vi "Write Discrete Inputs.vi"(8 "error in (no error)":errorcluster, 9 "input values":bool[](array[boolean]), 10 "starting address":u16, 11 "standard data model in":refnum<class "ICPCON ET Data Model.lvclass">) -> (0 "error out":errorcluster, 3 "standard data model out":refnum<class "ICPCON ET Data Model.lvclass">)   [LabVIEW 2021, in "ICPCON ET Data Model.lvclass"]
doc: "Writes the values of multiple discrete input values in series, starting at address M."
uses:
  ICPCON ET Data Model.lvclass
  ICPCON ET Data Model.lvclass/ICPCON ET Data Model.ctl
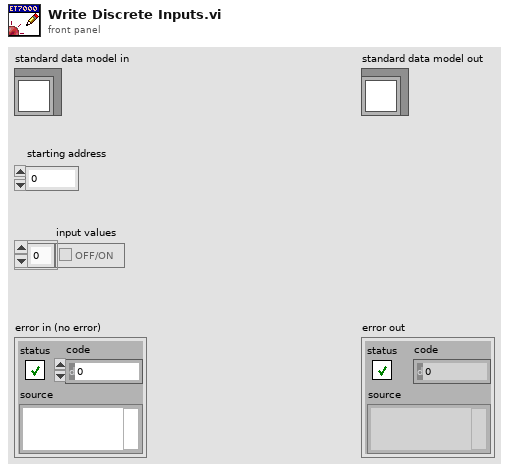
[diagram p1: front panel]
types:
  T1 = typedef "ICPCON ET Data Model.lvclass/Data Model.ctl" = cluster{"UTC":u64, "DI":bool[], "DO":bool[], "IR":u16[], "HR":u16[], "ES":u8}
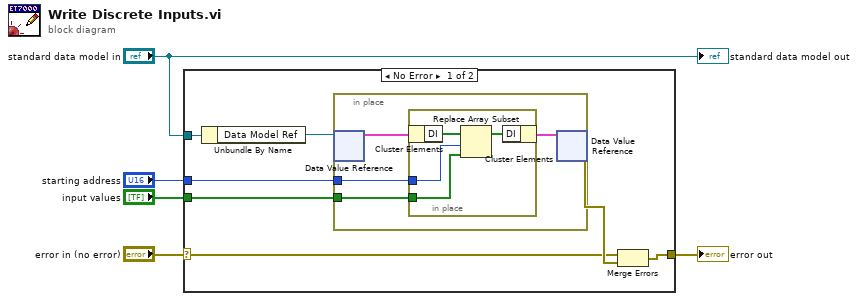
[diagram p0: block diagram]
diagram:
  n1 = case shown="No Error" "error in (no error)" {
    selector: "error in (no error)" -> [w6 w21]
    tunnel: "starting address" -> [w12 _]
    tunnel: "input values" -> [w11 _]
    tunnel: "standard data model in" -> [w10 _]
    tunnel: [w9 w21] -> w2
    frame No Error {
      n2 = Unbundle By Name(w10) -> ("Data Model Ref"=w8:refnum<data-value>)
      n3 = in-place {
        in-place-border: w12 -> [w16]
        in-place-border: w11 -> [w15]
        n4 = in-place-dvr #1(w8) -> (w14:T1)  [unwired: 1 out]
        n5 = in-place {
          in-place-border: w16 -> [w20]
          in-place-border: w15 -> [w19]
          n6 = in-place-cluster #2(w14) -> ("DI"=w18:bool[])
          n7 = Replace Array Subset(array=w18, new element=w19, index=w20) -> (w17:bool[])
          n8 = in-place-cluster #2("DI"=w17) -> (w13:T1)
        }
        n9 = in-place-dvr #1(w13) -> (w7:errorcluster)  [unwired: 1 out]
      }
      n10 = Merge Errors(w6, w7) -> (w9:errorcluster)
    }
    frame Error {
    }
  }
  "error out" <- w2
  "standard data model out" <- "standard data model in"
